vi "Quadratic Programming.vi"(6 "stopping Criteria":T2, 7 "UB":dbl=1000000.0 format="%#_13g", 9 "LB":dbl=-1000000.0 format="%#_13g", 10 "Desired Force Matrix":T1, 11 "Jacobian":T1) -> (1 "Boolean":bool, 2 "Q":T1=[[2.0000000000000004, 0.2948894830594344, -1.9987156983704204], [0.2948894830594344, 2.0, -0.22382057154195537], [-1.9987156983704204, -0.22382057154195537, 2.0000000000000004]], 3 "c":T1=[[-10.509026510636803], [-9.557653838992561], [10.212163924365424]], 4 "minimum":dbl[](array[numeric]))   [LabVIEW 2021]
uses:
  <vilib>/Analysis/Matrix/Datatypes/RealMatrix.ctl
  <vilib>/gmath/NumericalOptimization/stopping criteria.ctl
  <vilib>/Analysis/baseanly.llb/Real A x B.vi
  <vilib>/Analysis/Matrix/Numeric/Multiply/Multiply - RM,R.vi
  <vilib>/Analysis/Matrix/Numeric/Conversions/Matrix To Array - RM.vi
  <vilib>/gmath/NumericalOptimization/Quadratic Programming AS.vi
  <vilib>/Analysis/NI_AALBase.lvlib
  <vilib>/Analysis/Matrix/NI_Matrix.lvlib
  <vilib>/gmath/NI_Gmath.lvlib
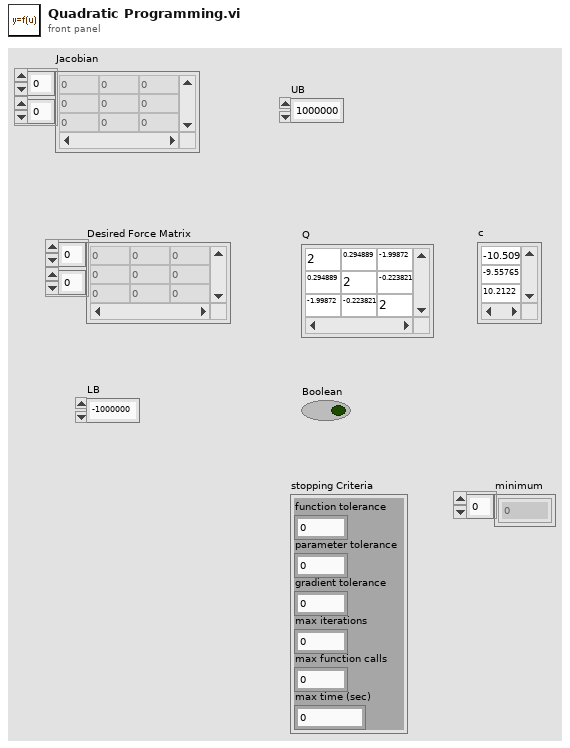
[diagram p1: front panel]
types:
  T1 = typedef "NI_Matrix.lvlib/RealMatrix.ctl" = dbl[][]
  T2 = typedef "NI_Gmath.lvlib/stopping criteria.ctl" = cluster{"function tolerance":dbl, "parameter tolerance":dbl, "max iterations":i32, "max function calls":i32, "gradient tolerance":dbl, "max time (sec)":dbl}
  T3 = cluster{"Real 2D Array":dbl[][], "Real 2D Array":dbl[]}
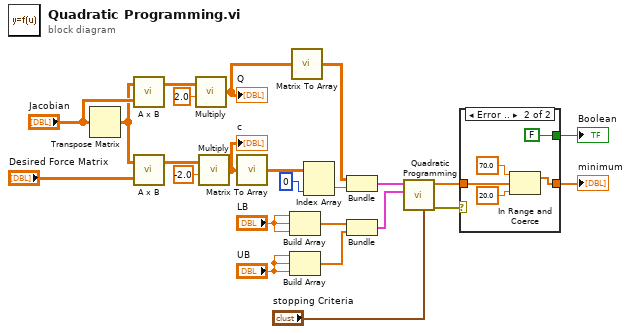
[diagram p0: block diagram]
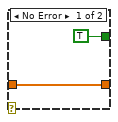
[diagram p2: hidden frame]
diagram:
  n1 = Transpose Matrix(1:"Jacobian") -> (0:w1:T1)
  n2 = call-poly <vilib>:"A x B.vi"("B"="Jacobian", "A"=w1) -> ("A x B"=w14:T1)  [unwired: 1 out]
  n3 = call-poly <vilib>:"A x B.vi"("B"="Desired Force Matrix", "A"=w1) -> ("A x B"=w16:T1)  [unwired: 1 out]
  n4 = call-poly <vilib>:"Multiply.vi"("Real Scalar c"=2.0 ("y"), "Real Matrix A"=w14) -> ("A * c"=w11:T1)
  "Q" <- w11
  n5 = call-poly <vilib>:"Multiply.vi"("Real Scalar c"=-2.0 ("y"), "Real Matrix A"=w16) -> ("A * c"=w12:T1)
  "c" <- w12
  n6 = call-poly <vilib>:"Matrix To Array.vi"("Real Matrix"=w12) -> ("Real 2D Array"=w18:dbl[][])
  n7 = Build Array("LB", "LB", "LB") -> (w21:dbl[])
  n8 = Build Array("UB", "UB", "UB") -> (w22:dbl[])
  n9 = call-poly <vilib>:"Matrix To Array.vi"("Real Matrix"=w11) -> ("Real 2D Array"=w17:dbl[][])
  n10 = Index Array(array=w18, index (col)=0 ("index")) -> (element=w19:dbl[])  [unwired: 1 in]
  n11 = Bundle("Real 2D Array"=w17, "Real 2D Array"=w19) -> (w20:T3)  [unwired: 1 in]
  n12 = Bundle(w21, w22) -> (w23:cluster{dbl[], dbl[]})  [unwired: 1 in]
  n13 = call-poly <vilib>:"Quadratic Programming.vi"("stopping criteria"="stopping Criteria", "parameter bounds"=w23, "objective function"=w20) -> ("error out"=w5:errorcluster, "minimum"=w7:dbl[])  [unwired: 5 in, 2 out]
  n14 = case shown="Error .." w5 {
    tunnel: [w25 w28] -> w10
    tunnel: [TRUE ("Boolean") FALSE ("Boolean")] -> w6
    tunnel: w7 -> [w25 w27]
    frame No Error {
    }
    frame Error {
      n15 = In Range and Coerce(upper limit=70.0 ("y"), x=w27, lower limit=20.0 ("y")) -> (coerced(x)=w28:dbl[])  [unwired: 1 out]
    }
  }
  "minimum" <- w10
  "Boolean" <- w6
